vi "Configure Class.vi"(5 "Standard (1)":i32=1, 6 "Type (0: Open)":u16(ring) items=["Open", "Short", "Load", "Thru", "Gain Phase Open", "Gain Phase Short", "Gain Phase Load", "Gain Phase Through"], 7 "Channel (1)":i32=1, 8 "error in (no error)":errorcluster, 9 "Port 2 (1)":i32=1, 10 "Port 1 (1)":i32=1, 11 "VISA resource name":refnum<visa-resource-name>) -> (0 "error out":errorcluster, 3 "VISA resource name out":refnum<visa-resource-name>)   [LabVIEW 2012, in "Tektronix TTR500 Series.lvlib"]
doc: "This VI configures calibration kit class."
uses:
  <instrlib>/Tektronix TTR500 Series/Tektronix TTR500 Series.lvlib
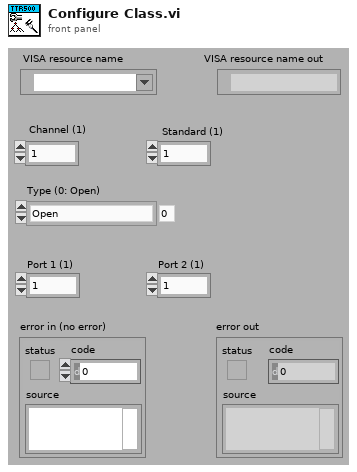
[diagram p1: front panel]
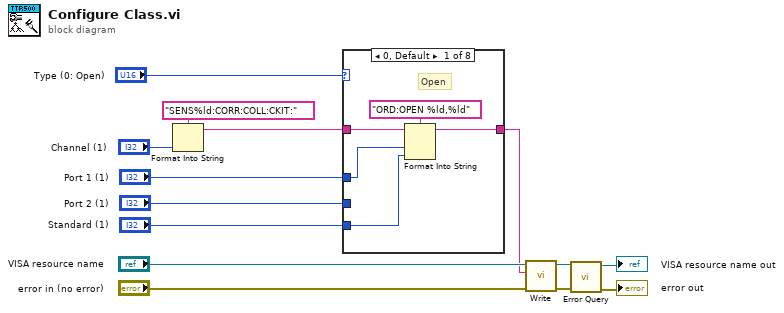
[diagram p0: block diagram]
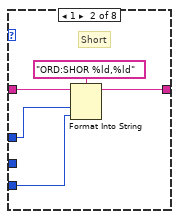
[diagram p2: hidden frame]
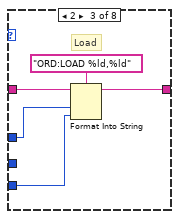
[diagram p3: hidden frame]
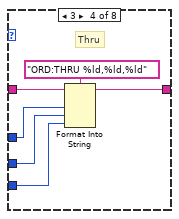
[diagram p4: hidden frame]
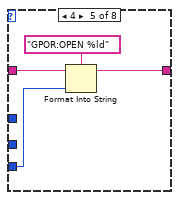
[diagram p5: hidden frame]
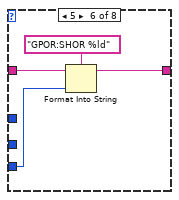
[diagram p6: hidden frame]
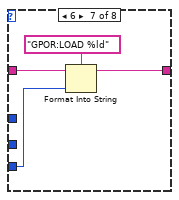
[diagram p7: hidden frame]
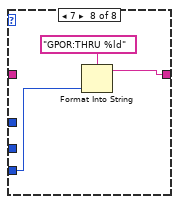
[diagram p8: hidden frame]
diagram:
  n1 = Format Into String(format string="SENS%ld:CORR:COLL:CKIT:", "Channel (1)") -> (resulting string=w9:string)  [unwired: 2 in, 1 out]
  n2 = case shown="0, Default" "Type (0: Open)" {
    tunnel: w9 -> [w18 w23 w28 w34 w38 w42 w46 _]
    tunnel: "Port 1 (1)" -> [w17 w22 w27 w33 _ _ _ _]
    tunnel: "Port 2 (1)" -> [_ _ _ w31 _ _ _ _]
    tunnel: [w16 w21 w26 w32 w37 w41 w45 w49] -> w5
    tunnel: "Standard (1)" -> [w15 w20 w25 w30 w36 w40 w44 w48]
    frame 0, Default {
      # "Open"
      n3 = Format Into String(format string="ORD:OPEN %ld,%ld", initial string=w18, w17, w15) -> (resulting string=w16:string)  [unwired: 1 in, 1 out]
    }
    frame 1 {
      # "Short"
      n4 = Format Into String(format string="ORD:SHOR %ld,%ld", initial string=w23, w22, w20) -> (resulting string=w21:string)  [unwired: 1 in, 1 out]
    }
    frame 2 {
      # "Load"
      n5 = Format Into String(format string="ORD:LOAD %ld,%ld", initial string=w28, w27, w25) -> (resulting string=w26:string)  [unwired: 1 in, 1 out]
    }
    frame 3 {
      # "Thru"
      n6 = Format Into String(format string="ORD:THRU %ld,%ld,%ld", initial string=w34, w33, w31, w30) -> (resulting string=w32:string)  [unwired: 1 in, 1 out]
    }
    frame 4 {
      n7 = Format Into String(format string="GPOR:OPEN %ld", initial string=w38, w36) -> (resulting string=w37:string)  [unwired: 1 in, 1 out]
    }
    frame 5 {
      n8 = Format Into String(format string="GPOR:SHOR %ld", initial string=w42, w40) -> (resulting string=w41:string)  [unwired: 1 in, 1 out]
    }
    frame 6 {
      n9 = Format Into String(format string="GPOR:LOAD %ld", initial string=w46, w44) -> (resulting string=w45:string)  [unwired: 1 in, 1 out]
    }
    frame 7 {
      n10 = Format Into String(format string="GPOR:THRU %ld", w48) -> (resulting string=w49:string)  [unwired: 2 in, 1 out]
    }
  }
  n11 = call <instrlib>:"Write.vi"("error in (no error)"="error in (no error)", "String ()"=w5, "VISA resource name"="VISA resource name") -> ("error out"=w3:errorcluster, "VISA resource name out"=w4:refnum<visa-resource-name>)  [unwired: 6 in, 1 out]
  n12 = call <instrlib>:"Error Query.vi"("error in (no error)"=w3, "VISA resource name"=w4) -> ("error out"=→"error out":errorcluster, "VISA resource name out"=→"VISA resource name out":refnum<visa-resource-name>)  [unwired: 6 in, 2 out]
